vi "11. FGV Message check.vi"(0 "VISA resource name":refnum<visa-resource-name>="COM3", 11 "error in (no error)":errorcluster) -> (3 "Err":i32, 4 "Machine":i32, 6 "Cmd":string, 8 "Cnt":u32, 10 "Data":i32[](array[numeric]), 15 "error out":errorcluster)   [LabVIEW 2014]
panel:
  out "Cksum":u32
  # "01 30 31 54 59 30 30 36 45 04"
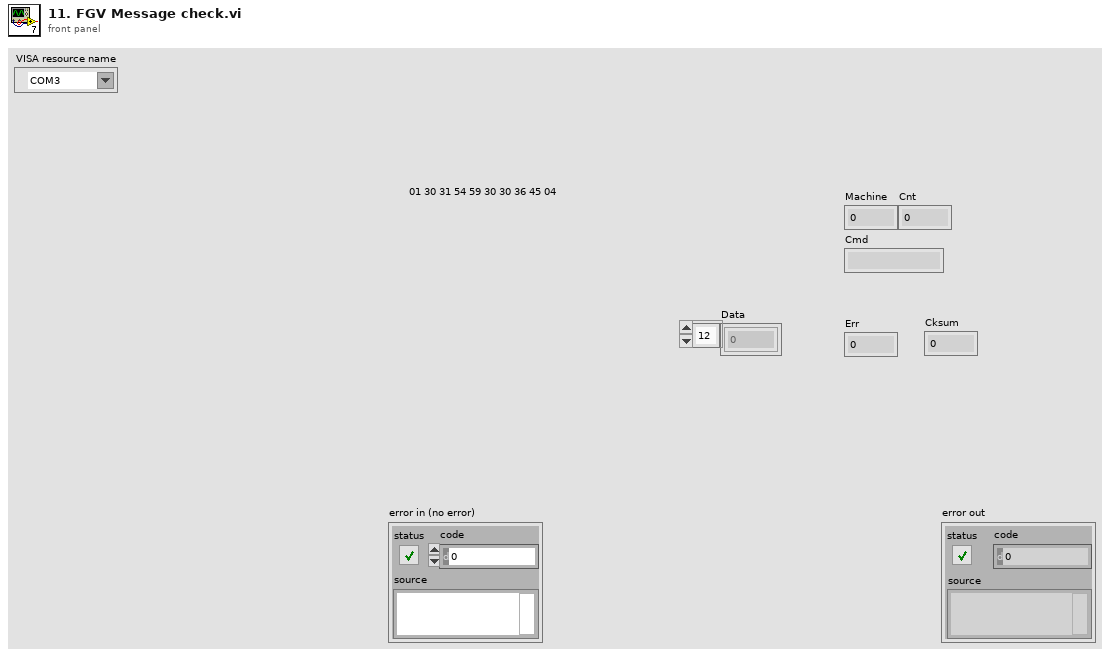
[diagram p1: front panel]
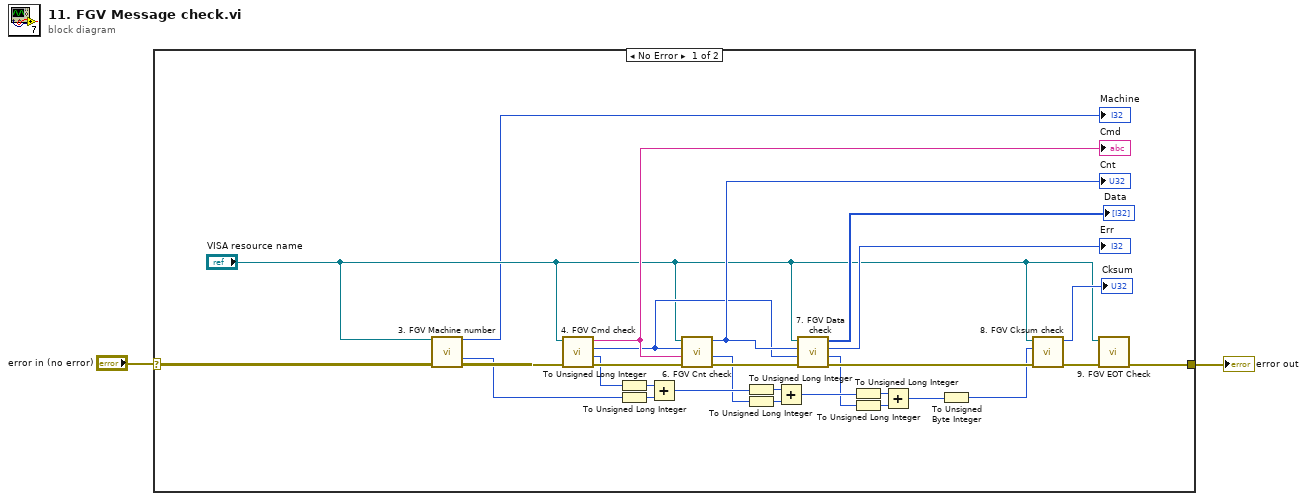
[diagram p0: block diagram]
diagram:
  n1 = case shown="No Error" "error in (no error)" {
    selector: "error in (no error)" -> [w7 w32]
    tunnel: [w8 w32] -> w1
    frame No Error {
      n2 = call "3. FGV Machine number.vi"("VISA resource name"="VISA resource name", "error in (no error)"=w7) -> ("Machine"=→"Machine":i32, "Checksum"=w3:u32, "error out"=w4:errorcluster)  [unwired: 11 in]
      n3 = call "4. FGV Cmd check.vi"("error in (no error)"=w4, "VISA resource name"="VISA resource name") -> ("error out"=w31:errorcluster, "Checksum"=w24:u32, "Command type (ACK, NACK, Normal)"=w11:i32, "Command"=w14:string)  [unwired: 6 in]
      "Cmd" <- w14
      n4 = To Unsigned Long Integer(number=w24) -> (unsigned 32bit integer=w26:u32)
      n5 = To Unsigned Long Integer(number=w3) -> (unsigned 32bit integer=w25:u32)
      n6 = Add(x=w26, y=w25) -> (x+y=w21:u32)
      n7 = call "6. FGV Cnt check.vi"("error in (no error)"=w31, "Command"=w14, "Command type (0 = Normal, 1= ACK, 2 = NACK)"=w11, "VISA resource name"="VISA resource name") -> ("error out"=w30:errorcluster, "Checksum"=w20:u32, "Cnt"=w12:u32)  [unwired: 5 in]
      "Cnt" <- w12
      n8 = To Unsigned Long Integer(number=w21) -> (unsigned 32bit integer=w23:u32)
      n9 = To Unsigned Long Integer(number=w20) -> (unsigned 32bit integer=w22:u32)
      n10 = Add(x=w23, y=w22) -> (x+y=w17:u32)
      n11 = call "7. FGV Data check.vi"("error in (no error)"=w30, "cmd type (CMD = 0, ACK = 1, NAK = 2)"=w11, "Cnt"=w12, "VISA resource name"="VISA resource name") -> ("error out"=w29:errorcluster, "Checksum"=w16:u32, "Error"=→"Err":i32, "Data"=→"Data":i32[])  [unwired: 4 in]
      n12 = To Unsigned Long Integer(number=w17) -> (unsigned 32bit integer=w19:u32)
      n13 = To Unsigned Long Integer(number=w16) -> (unsigned 32bit integer=w18:u32)
      n14 = Add(x=w19, y=w18) -> (x+y=w15:u32)
      n15 = To Unsigned Byte Integer(number=w15) -> (unsigned 8bit integer=w10:u8)
      n16 = call "8. FGV Cksum check.vi"("error in (no error)"=w29, "Calculated cksum"=w10, "VISA resource name"="VISA resource name") -> ("error out"=w28:errorcluster, "Cksum"=→"Cksum":u32)  [unwired: 7 in]
      n17 = call "9. FGV EOT Check.vi"("error in (no error)"=w28, "VISA resource name"="VISA resource name") -> ("error out"=w8:errorcluster)  [unwired: 8 in, 1 out]
    }
    frame Error {
    }
  }
  "error out" <- w1
